vi "Translate_PolarVector.vi"(7 "Translation Type":T1, 8 "error in (no error)":errorcluster, 10 "PolarVector in 2":refnum<class "PolarVector.lvclass">, 11 "PolarVector in":refnum<class "PolarVector.lvclass">) -> (0 "error out":errorcluster, 3 "PolarVector out":refnum<class "PolarVector.lvclass">)   [LabVIEW 2012, in "PolarVector.lvclass"]
doc: "Takes in two PolarVector objects and translation type. Translates the first by the second according to the translation type and outputs a new PolarVector object."
uses:
  PolarVector.lvclass
  TypeDefs/TranslationType.ctl
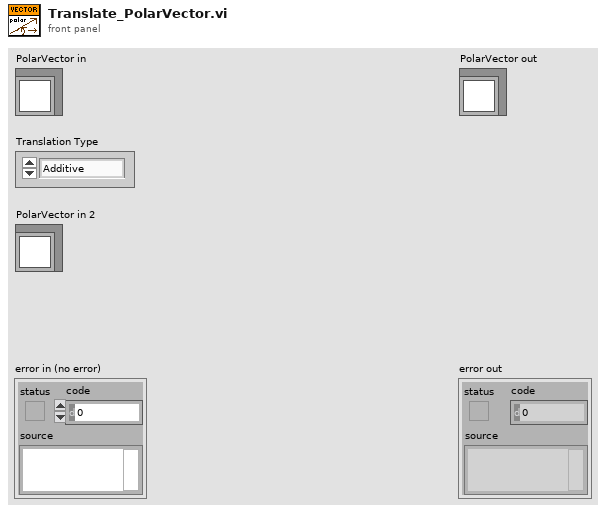
[diagram p1: front panel]
types:
  T1 = typedef "TranslationType.ctl" = enum16{"Additive", "Subtractive"}
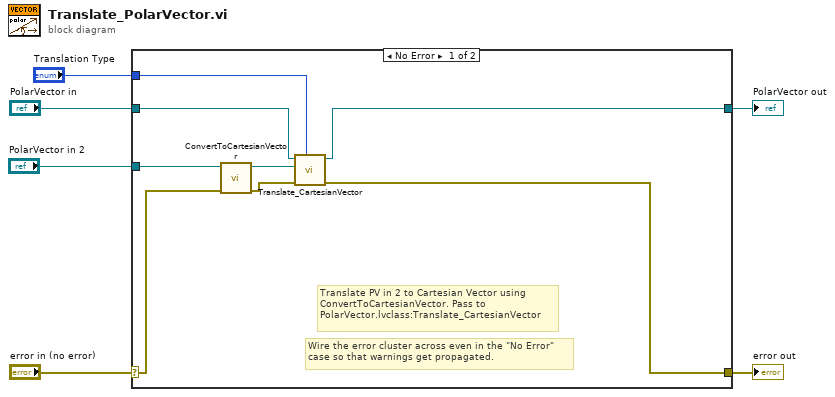
[diagram p0: block diagram]
diagram:
  n1 = case shown="No Error" "error in (no error)" {
    selector: "error in (no error)" -> [w10 w16]
    tunnel: [w7 w16] -> w5
    tunnel: [w8 w15] -> w3
    tunnel: "PolarVector in" -> [w13 w15]
    tunnel: "PolarVector in 2" -> [w14 _]
    tunnel: "Translation Type" -> [w12 _]
    frame No Error {
      # "Translate PV in 2 to Cartesian Vector using\nConvertToCartesianVector. Pass to \nPolarVector.lvclass:Translate_CartesianVector"
      # "Wire the error cluster across even in the \"No Error\"\ncase so that warnings get propagated."
      n2 = call "ConvertToCartesianVector.vi"("error in (no error)"=w10, "PolarVector in"=w14) -> ("error out"=w9:errorcluster, "CartesianVector.lvclass"=w11:refnum<class "CartesianVector.lvclass">)  [unwired: 8 in]
      n3 = call "Translate_CartesianVector.vi"("Translation Type"=w12, "error in (no error)"=w9, "CartesianVector.lvclass"=w11, "PolarVector in"=w13) -> ("error out"=w7:errorcluster, "PolarVector out"=w8:refnum<class "PolarVector.lvclass">)  [unwired: 6 in]
    }
    frame Error {
    }
  }
  "error out" <- w5
  "PolarVector out" <- w3
